vi "ziSweepGenerator.vi"(0 "Steps (#)":i32=2, 1 "Start (Hz)":dbl=10.0 format="%#_12p", 2 "Harmonic (1)":i32=1, 3 "Min 1-w Damping (40dB)":dbl=40.0, 5 "Order (4)":i32=4, 7 "Bandwith (-1=auto)":dbl=-1.0 format="%#_12p", 9 "Log Sweep (true)":bool=TRUE, 11 "Precision (Low)":i32(ring) items=["Low", "Medium", "High"], 12 "Stop (Hz)":dbl=10000.0 format="%#_12p", 13 "Mode":enum16{"Spectrum", "FRA"}(ring)) -> (8 "Sweep Sequence (F (Hz), BW (Hz), TC(s), Time(s))":dbl[][](array[numeric]) format="%#_6p", 10 "Omega-component limited":bool, 15 "Coverage Gaps":bool)   [LabVIEW 2018, in "Zurich Instruments LabOne.lvlib"]
doc: "---Obsolete---\n(Please, use the sweeper module)\nCaluculate frequencies, filter settings and settle times for a frequency sweep.\n\n<b>Coverage Gaps</b>: when true, the requency steps are too large to be covered even with max bandwidth of the demodulator. Only a problem when used as spectrum analyzer, no problem when used as a network analyzer."
uses:
  Zurich Instruments LabOne.lvlib
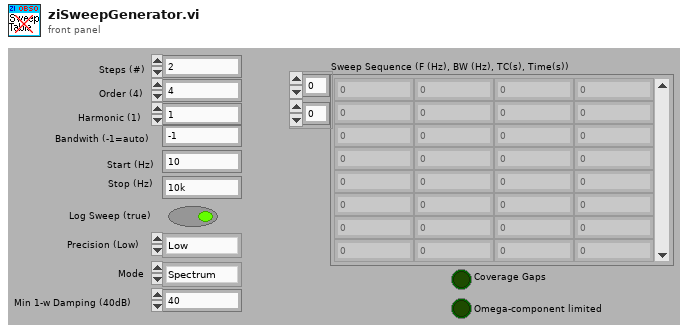
[diagram p1: front panel]
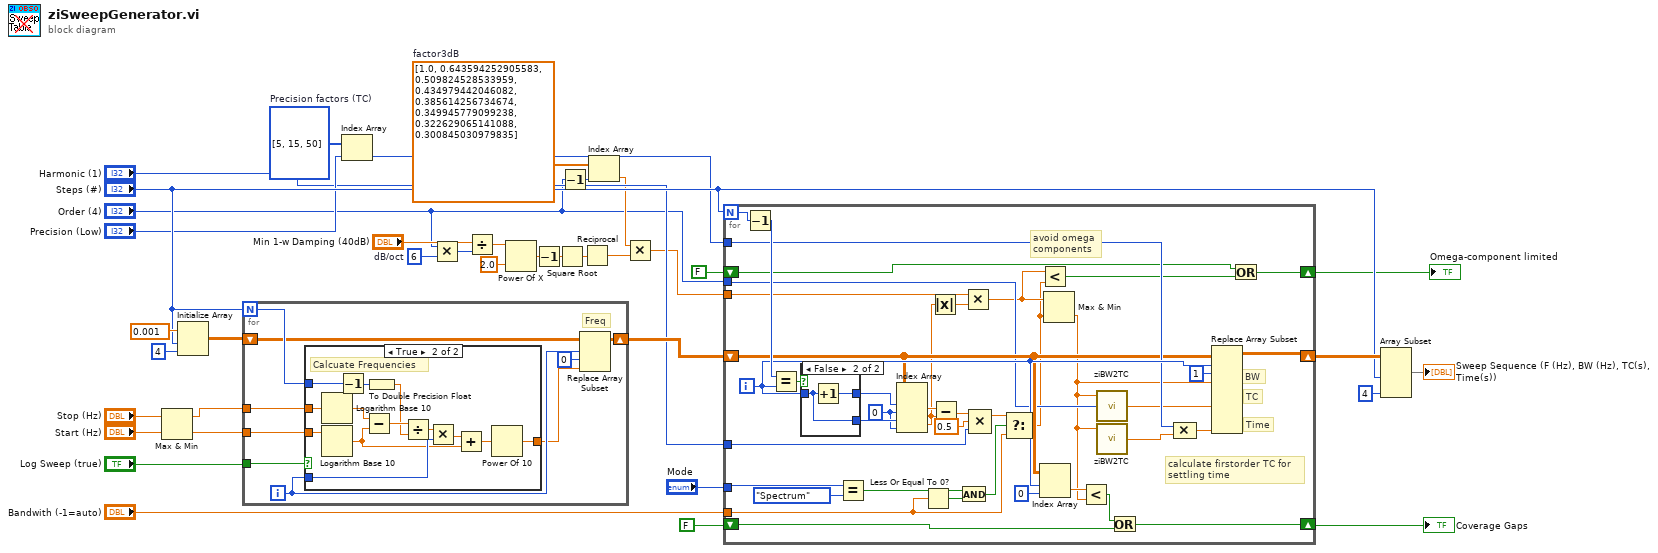
[diagram p0: block diagram]
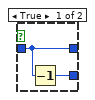
[diagram p2: hidden frame]
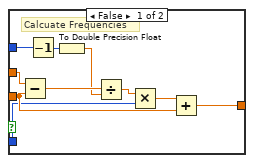
[diagram p3: hidden frame]
diagram:
  w5 = dbl[] [1.0, 0.643594252905583, 0.509824528533959, 0.434979442046082, 0.385614256734674, 0.349945779099238, 0.322629065141088, 0.300845030979835]  # factor3dB
  w14 = 6  # dB/oct
  w21 = i32[] [5, 15, 50]  # Precision factors (TC)
  n1 = Max & Min(x="Stop (Hz)", y="Start (Hz)") -> (max(x,y)=w26:dbl, min(x,y)=w25:dbl)
  n2 = Initialize Array(0.001 ("element"), "Steps (#)", 4 ("dimension size")) -> (w35:dbl[][])
  n3 = for {
    N: "Steps (#)" -> [w44]
    tunnel: w25 -> [w45]
    tunnel: w26 -> [w46]
    shift-right: [w39] -> w34
    shift-left: w35 -> [w38]
    tunnel: "Log Sweep (true)" -> [w42]
    i -> [w41]
    # "Freq"
    n4 = case shown="True" w42 {
      tunnel: w46 -> [w56 w68]
      tunnel: w45 -> [w52 w69]
      tunnel: w44 -> [w49 w58]
      tunnel: w41 -> [w51 w66]
      tunnel: [w50 w62] -> w40
      frame False {
        # "Calcuate Frequencies"
        n5 = Subtract(x=w56, y=w52) -> (x-y=w55:dbl)
        n6 = Decrement(x=w49) -> (x-1=w48:i32)
        n7 = To Double Precision Float(number=w48) -> (double precision float=w47:dbl)
        n8 = Divide(x=w55, y=w47) -> (x/y=w54:dbl)
        n9 = Multiply(x=w54, y=w51) -> (x*y=w53:dbl)
        n10 = Add(x=w53, y=w52) -> (x+y=w50:dbl)
      }
      frame True {
        # "Calcuate Frequencies"
        n11 = Logarithm Base 10(1:w68) -> (0:w61:dbl)
        n12 = Logarithm Base 10(1:w69) -> (0:w60:dbl)
        n13 = Decrement(x=w58) -> (x-1=w59:i32)
        n14 = Subtract(x=w61, y=w60) -> (x-y=w67:dbl)
        n15 = To Double Precision Float(number=w59) -> (double precision float=w57:dbl)
        n16 = Divide(x=w67, y=w57) -> (x/y=w65:dbl)
        n17 = Multiply(x=w65, y=w66) -> (x*y=w64:dbl)
        n18 = Add(x=w64, y=w60) -> (x+y=w63:dbl)
        n19 = Power Of 10(x=w63) -> (10^x=w62:dbl)
      }
    }
    n20 = Replace Array Subset(array=w38, new element=w40, index (row)=w41, index (col)=0 ("disabled index (col)")) -> (w39:dbl[][])
  }
  n21 = Index Array(array=w21, index="Precision (Low)") -> (element=w19:i32)
  n22 = Multiply(x="Order (4)", y=w14) -> (x*y=w15:i32)
  n23 = Divide(x="Min 1-w Damping (40dB)", y=w15) -> (x/y=w13:dbl)
  n24 = Power Of X(1:2.0 ("x"), 2:w13) -> (0:w11:dbl)
  n25 = Decrement(x=w11) -> (x-1=w9:dbl)
  n26 = Square Root(x=w9) -> (sqrt(x)=w6:dbl)
  n27 = Decrement(x="Order (4)") -> (x-1=w1:i32)
  n28 = Reciprocal(x=w6) -> (1/x=w10:dbl)
  n29 = Index Array(array=w5, index=w1) -> (element=w3:dbl)
  n30 = Multiply(x=w3, y=w10) -> (x*y=w4:dbl)
  n31 = for {
    N: "Steps (#)" -> [w107]
    shift-right: [w108] -> w33
    shift-left: w34 -> [w88]
    tunnel: "Order (4)" -> [w86]
    tunnel: w19 -> [w92]
    tunnel: "Bandwith (-1=auto)" -> [w100]
    shift-right: [w96] -> w27
    shift-left: FALSE -> [w94]
    tunnel: "Harmonic (1)" -> [w87]
    tunnel: "Mode" -> [w80]
    tunnel: w4 -> [w77]
    shift-right: [w72] -> w7
    shift-left: FALSE -> [w71]
    i -> [w93]
    w90 = 0 ("disabled index (col)")
    # "avoid omega\ncomponents"
    # "calculate firstorder TC for\nsettling time"
    # "TC"
    # "Time"
    # "BW"
    n32 = Decrement(x=w107) -> (x-1=w106:i32)
    n33 = Equal?(x=w106, y=w93) -> (x = y?=w105:bool)
    n34 = case shown="False" w105 {
      tunnel: w93 -> [w110 w113]
      tunnel: [w111 w113] -> w91
      tunnel: [w110 w112] -> w102
      frame True {
        n35 = Decrement(x=w110) -> (x-1=w111:i32)
      }
      frame False {
        n36 = Increment(x=w113) -> (x+1=w112:i32)
      }
    }
    n37 = Equal?(x=w80, y=enum16{"Spectrum", "FRA"}."Spectrum") -> (x = y?=w78:bool)
    n38 = Index Array(array=w88, index (row) #1=w102, index (col) #1=w90, index (row) #2=w91, index (col) #2=w90) -> (element #1=w83:dbl, element #2=w70:dbl)
    n39 = Less Or Equal To 0?(x=w100) -> (x <= 0?=w99:bool)
    n40 = Absolute Value(x=w70) -> (abs(x)=w76:dbl)
    n41 = Subtract(x=w83, y=w70) -> (x-y=w103:dbl)
    n42 = And(x=w78, y=w99) -> (x .and. y?=w81:bool)
    n43 = Multiply(x=w77, y=w76) -> (x*y=w75:dbl)
    n44 = Compound Arithmetic op=MULTIPLY(w103, 0.5 ("x-y"), w87) -> (w101:dbl)
    n45 = Select(t=w101, s=w81, f=w100) -> (s? t:f=w74:dbl)
    n46 = Less?(x=w75, y=w74) -> (x < y?=w73:bool)
    n47 = Index Array(array=w88, index (row)=w93, index (col)=0 ("disabled index (col)")) -> (element=w97:dbl)
    n48 = Max & Min(x=w75, y=w74) -> (min(x,y)=w82:dbl)  [unwired: 1 out]
    n49 = Less?(x=w97, y=w82) -> (x < y?=w95:bool)
    n50 = call "ziBW2TC.vi"("Order (1)"=w86, "BW (Hz)"=w82) -> ("TC (s)"=w85:dbl)  [unwired: 1 in]
    n51 = call "ziBW2TC.vi"("BW (Hz)"=w82) -> ("TC (s)"=w84:dbl)  [unwired: 2 in]
    n52 = Or(x=w95, y=w94) -> (x .or. y?=w96:bool)
    n53 = Compound Arithmetic op=MULTIPLY(w92, w84) -> (w89:dbl)
    n54 = Replace Array Subset(array=w88, new element #1=w82, index (row) #1=w93, index (col) #1=1 ("disabled index (col)"), new element #2=w85, new element #3=w89) -> (w108:dbl[][])  [unwired: 4 in]
    n55 = Or(x=w71, y=w73) -> (x .or. y?=w72:bool)
  }
  "Coverage Gaps" <- w27
  "Omega-component limited" <- w7
  n56 = Array Subset(array=w33, length (row)="Steps (#)", length (col)=4 ("length")) -> (→"Sweep Sequence (F (Hz), BW (Hz), TC(s), Time(s))":dbl[][])  [unwired: 2 in]
